vi "Launch TCP Server Engine.vi"(8 "error in (no error)":errorcluster, 9 "User Events":T1, 10 "Port (0)":i32, 11 "Service Name":string) -> (0 "error out":errorcluster)   [LabVIEW 2016, in "SLL Easy API via TCP.lvclass"]
uses:
  SLL Easy API via TCP.lvclass
  _Typedefs/User Events to TCP Engine.ctl
  _Typedefs/TCP Event Data.ctl
  TCP Server Engine.vi
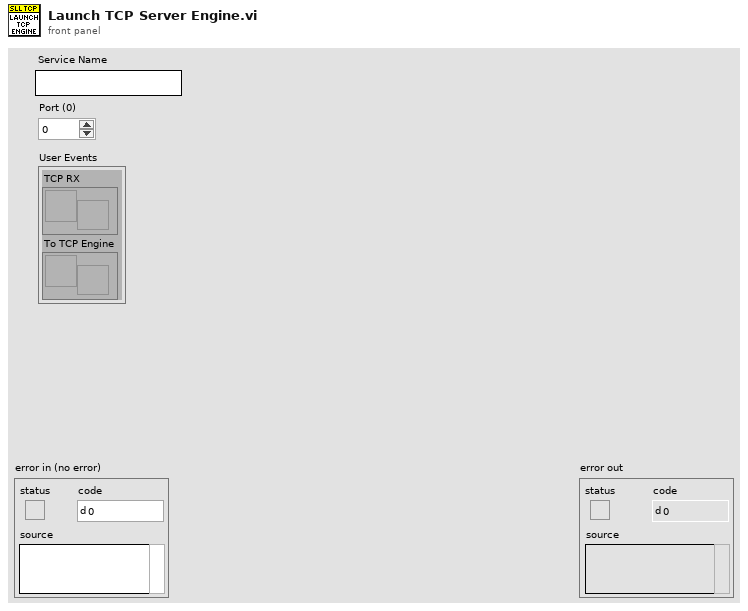
[diagram p1: front panel]
types:
  T1 = typedef "SLL Easy API via TCP.lvclass/User Events to TCP Engine.ctl" = cluster{"TCP RX":refnum<user-event>, "To TCP Engine":refnum<user-event>}
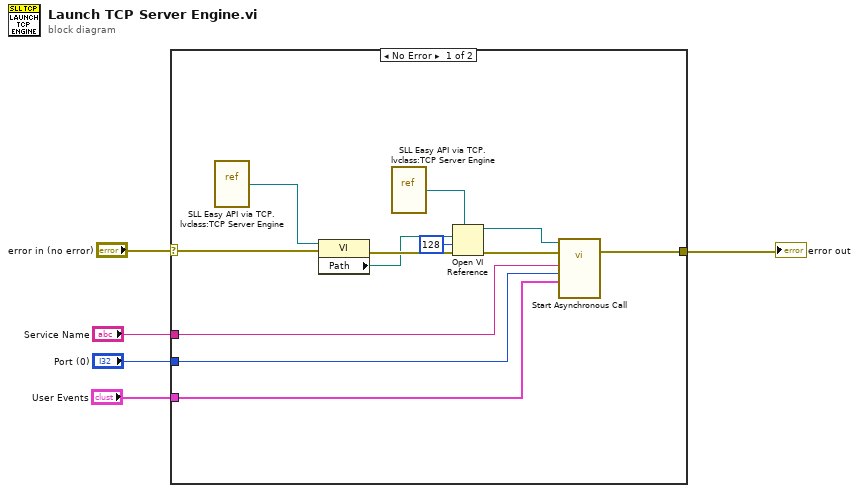
[diagram p0: block diagram]
diagram:
  n1 = case shown="No Error" "error in (no error)" {
    selector: "error in (no error)" -> [w14 w18]
    tunnel: [w10 w18] -> w4
    tunnel: "Service Name" -> [w9 _]
    tunnel: "Port (0)" -> [w8 _]
    tunnel: "User Events" -> [w7 _]
    frame No Error {
      n2 = vi-ref "SLL Easy API via TCP.lvclass:TCP Server Engine.vi"() -> (w17:refnum<vi>)
      n3 = property class="VI"(reference=w17, error in=w14) -> (error out=w16:errorcluster, "Path"=w15:path)  [unwired: 1 out]
      n4 = vi-ref "SLL Easy API via TCP.lvclass:TCP Server Engine.vi"() -> (w13:refnum<vi>)
      n5 = Open VI Reference(type specifier VI Refnum (for type only)=w13, vi path=w15, options=128, error in (no error)=w16) -> (vi reference=w12:refnum<vi>, error out=w11:errorcluster)  [unwired: 2 in]
      n6 = call-by-ref "Start Asynchronous Call"(reference=w12, error in=w11, "User Events"=w7, "Port (0)"=w8, "Service Name"=w9) -> (error out=w10:errorcluster)  [unwired: 8 in, 2 out]
    }
    frame Error {
    }
  }
  "error out" <- w4
